vi "row or col find.vi"(1 "row or col":i32[](array[numeric]), 2 "1~9 input":i32[](array[numeric])) -> (0 "1~9 output":i32[](array[numeric]))   [LabVIEW 2014]
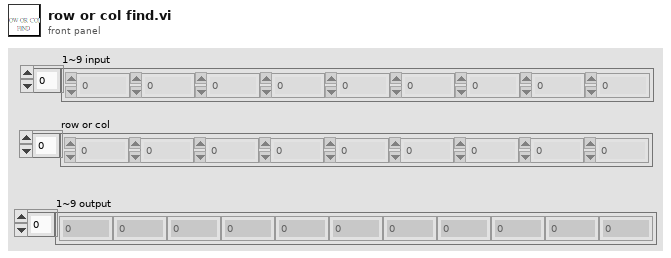
[diagram p1: front panel]
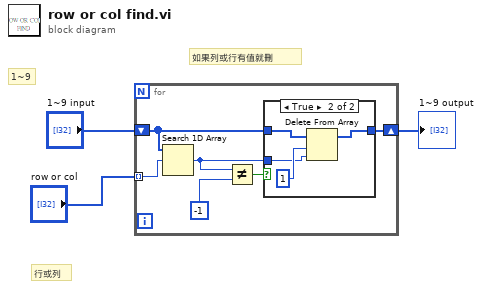
[diagram p0: block diagram]
diagram:
  # "如果列或行有值就刪"
  # "行或列"
  # "1~9"
  n1 = for {
    tunnel: "row or col" -> [w9] mode=indexing
    shift-right: [w5] -> w1
    shift-left: "1~9 input" -> [w4]
    n2 = Search 1D Array(1D array=w4, element=w9) -> (index of element=w7:i32)  [unwired: 1 in]
    n3 = Not Equal?(x=w7, y=-1) -> (x != y?=w6:bool)
    n4 = case shown="True" w6 {
      tunnel: w4 -> [w10 w14]
      tunnel: w7 -> [_ w12]
      tunnel: [w10 w11] -> w5
      frame False {
      }
      frame True {
        n5 = Delete From Array(array=w14, length=1, index=w12) -> (array with subset deleted=w11:i32[])  [unwired: 1 out]
      }
    }
  }
  "1~9 output" <- w1
